vi "17.1.3 Classifier Training-Grayscale.vi"() -> ()   [LabVIEW 2016]
uses:
  <vilib>/vision/Classification.llb/IMAQ Classifier Nearest Neighbor Training Results.ctl
  <vilib>/vision/Classification.llb/IMAQ Classification Particle Classification options.ctl
  <vilib>/vision/Classification.llb/IMAQ Classification Particle AutoThreshold Options.ctl
  <vilib>/vision/Classification.llb/IMAQ Classifier Nearest Neighbor options.ctl
  <vilib>/vision/Classification.llb/IMAQ Classifier Write Options.ctl
  <vilib>/vision/NI_Vision_Development_Module.lvlib
panel:
  out "Class Distance Table":dbl[][](array[numeric]) format="%.2f"
  out "Training Results":T1[](array[typedef]) {"Standard Deviation" format="%.2f"}
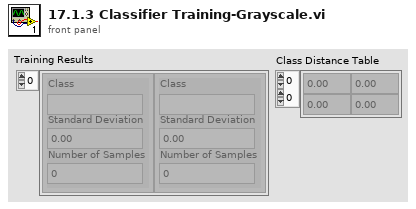
[diagram p1: front panel]
types:
  T1 = typedef "IMAQ Classifier Nearest Neighbor Training Results.ctl" = cluster{"Class":string, "Standard Deviation":sgl, "Number of Samples":i32}
  T2 = typedef "IMAQ Classifier Write Options.ctl" = i32
  T3 = typedef "IMAQ Classifier Nearest Neighbor options.ctl" = cluster{"Method":i32, "Metric":i32, "k":i32}
  T4 = typedef "IMAQ Classification Particle AutoThreshold Options.ctl" = cluster{"Method":i32, "Look For (Bright Objects)":u32, "Threshold Limits":cluster{"Lower value":sgl, "Upper value":sgl}}
  T5 = typedef "IMAQ Classification Particle Classification options.ctl" = cluster{"Scale Dependence":sgl, "Mirror Dependence":sgl}
  T6 = typedef "IMAQ Classifier Session.ctl" = refnum<k1>
  T7 = typedef "IMAQ Image.ctl" = refnum<image>
  T8 = typedef "ROI Descriptor" = cluster{"Global Rectangle":i32[], "Contours":cluster{"ID":enum32{"External", "Internal"}, "Type":u32, "Coordinates":i32[]}[]}
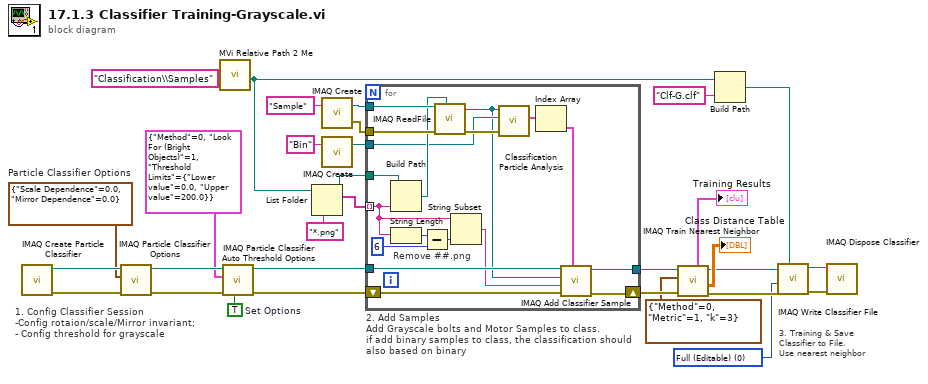
[diagram p0: block diagram]
diagram:
  w3 = T2 0 items=["Full (Editable)", "Compact (Not Editable)"] ("Write Options")
  w19 = TRUE  # Set Options
  w21 = T5 {"Scale Dependence"=0.0, "Mirror Dependence"=0.0}  # Particle Classifier Options
  # "3. Training & Save Classifier to File.\nUse nearest neighbor"
  # "2. Add Samples\nAdd Grayscale bolts and Motor Samples to class.\nif add binary samples to class, the classification should also based on binary"
  # "1. Config Classifier Session\n-Config rotaion/scale/Mirror invariant;\n- Config threshold for grayscale"
  n1 = call "IMAQ Create Particle Classifier"() -> ("error out"=w24:errorcluster, "Classifier Session"=w25:T6)  [unwired: 10 in]
  n2 = call "IMAQ Particle Classifier Options"("error in (no error)"=w24, "Particle Classifier Options"=w21, "Classifier Session"=w25) -> ("error out"=w22:errorcluster, "Classifier Session (dup)"=w23:T6)  [unwired: 6 in, 1 out]
  n3 = call "MVi Relative Path 2 Me.vi"("Relative Path"="Classification\\Samples") -> ("Appended Dir"=w8:path)  [unwired: 5 in, 1 out]
  n4 = call "IMAQ Particle Classifier Auto Threshold Options"("Get/Set Options? (Get)"=w19, "error in (no error)"=w22, "AutoThreshold Options In"=T4 {"Method"=0, "Look For (Bright Objects)"=1, "Threshold Limits"={"Lower value"=0.0, "Upper value"=200.0}}, "Classifier Session"=w23) -> ("error out"=w17:errorcluster, "Classifier Session (dup)"=w18:T6)  [unwired: 5 in, 1 out]
  n5 = List Folder(path=w8, pattern="*.png") -> (path out=w26:path, filenames=w29:string[])  [unwired: 2 in, 2 out]
  n6 = call "IMAQ Create"("Image Name"="Sample") -> ("Src"=w27:T7, "error out"=w9:errorcluster)  [unwired: 4 in]
  n7 = call "IMAQ Create"("Image Name"="Bin") -> ("Src"=w1:T7)  [unwired: 4 in, 1 out]
  n8 = for {
    tunnel: w29 -> [w43] mode=indexing
    tunnel: w18 -> [w46]
    tunnel: w27 -> [w42]
    tunnel: w26 -> [w44]
    shift-right: [w40] -> w15
    shift-left: w17 -> [w41]
    tunnel: [w39] -> w16
    tunnel: w9 -> [w38]
    tunnel: w1 -> [w34]
    # "Remove ##.png"
    n9 = Build Path(base path=w44, name or relative path=w43) -> (appended path=w37:path)
    n10 = String Length(string=w43) -> (length=w49:i32)
    n11 = Subtract(x=w49, y=6) -> (x-y=w47:i32)
    n12 = call "IMAQ ReadFile"("File Path"=w37, "error in (no error)"=w38, "Image"=w42) -> ("error out"=w36:errorcluster, "Image Out"=w32:T7)  [unwired: 4 in, 3 out]
    n13 = String Subset(string=w43, length (rest)=w47) -> (substring=w45:string)  [unwired: 1 in]
    n14 = call "Classification Particle Analysis.vi"("error in (no error)"=w36, "Image Dest"=w34, "Image Source"=w32) -> ("ROIs"=w35:T8[])  [unwired: 5 in, 3 out]
    n15 = Index Array(array=w35) -> (element=w33:T8)  [unwired: 1 in]
    n16 = call "IMAQ Add Classifier Sample"("ROI Descriptor"=w33, "error in (no error)"=w41, "Class"=w45, "Image"=w32, "Classifier Session"=w46) -> ("error out"=w40:errorcluster, "Classifier Session (dup)"=w39:T6)  [unwired: 4 in, 1 out]
  }
  n17 = call "IMAQ Train Nearest Neighbor"("error in (no error)"=w15, "Nearest Neighbor Options"=T3 {"Method"=0, "Metric"=1, "k"=3}, "Classifier Session"=w16) -> ("error out"=w10:errorcluster, "Class Distance Table"=→"Class Distance Table":dbl[][], "Classifier Session (dup)"=w11:T6, "Training Results"=→"Training Results":T1[])  [unwired: 5 in]
  n18 = Build Path(base path=w8, name or relative path="Clf-G.clf" ("pattern")) -> (appended path=w6:path)
  n19 = call "IMAQ Write Classifier File"("File Path"=w6, "error in (no error)"=w10, "Write Options"=w3, "Classifier Session"=w11) -> ("error out"=w5:errorcluster, "Classifier Session (dup)"=w4:T6)  [unwired: 6 in]
  n20 = call "IMAQ Dispose Classifier"("error in (no error)"=w5, "Classifier Session"=w4) -> ()  [unwired: 9 in, 1 out]
